vi "UNI_MAGFileToData.vi"(0 "spreadsheetData":string) -> (4 "names":string[](array[string]), 6 "settings":dbl[](array[numeric]) format="%.2f", 8 "polarities":i32[](array[numeric]), 10 "statuses":i32[](array[numeric]), 11 "allNames":bool, 12 "allSettings":bool, 13 "allPolarities":bool, 14 "allStatuses":bool, 15 "allRight":bool)   [LabVIEW 2014]
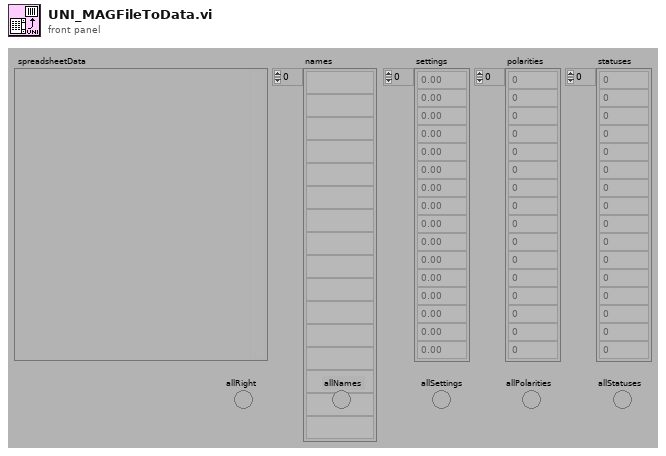
[diagram p1: front panel]
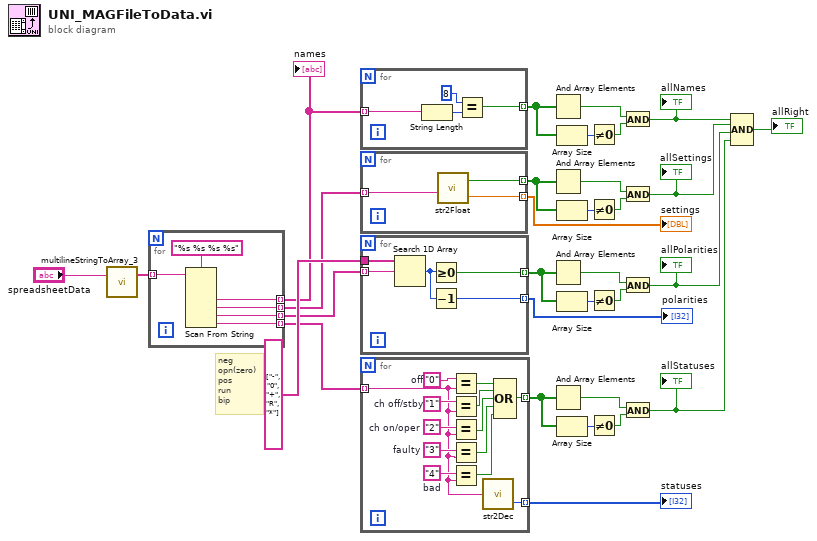
[diagram p0: block diagram]
diagram:
  # "neg\nopn(zero)\npos\nrun\nbip"
  n1 = call "multilineStringToArray_3.vi"("multilineString"="spreadsheetData") -> ("stringArray"=w15:string[])  [unwired: 1 in, 1 out]
  n2 = for {
    tunnel: w15 -> [w37] mode=indexing
    tunnel: [w35] -> w17 mode=indexing
    tunnel: [w34] -> w16 mode=indexing
    tunnel: [w33] -> w7 mode=indexing
    tunnel: [w32] -> w9 mode=indexing
    n3 = Scan From String(format string="%s %s %s %s", input string=w37) -> (output 1=w35:string, output 2=w34:string, output 3=w33:string, output 4=w32:string)  [unwired: 6 in, 3 out]
  }
  "names" <- w17
  n4 = for {
    tunnel: w17 -> [w41] mode=indexing
    tunnel: [w38] -> w19 mode=indexing
    n5 = String Length(string=w41) -> (length=w40:i32)
    n6 = Equal?(x=8, y=w40) -> (x = y?=w38:bool)
  }
  n7 = for {
    tunnel: w16 -> [w44] mode=indexing
    tunnel: [w43] -> w30 mode=indexing
    tunnel: [w42] -> w18 mode=indexing
    n8 = call "str2Float.vi"("string"=w44) -> ("is a floating"=w43:bool, "number"=w42:dbl)
  }
  "settings" <- w18
  n9 = for {
    tunnel: [w47] -> w24 mode=indexing
    tunnel: string[] ["-", "0", "+", "R", "*"] -> [w49]
    tunnel: w7 -> [w48] mode=indexing
    tunnel: [w45] -> w6 mode=indexing
    n10 = Search 1D Array(1D array=w49, element=w48) -> (index of element=w46:i32)  [unwired: 1 in]
    n11 = Greater Or Equal To 0?(x=w46) -> (x >= 0?=w47:bool)
    n12 = Decrement(x=w46) -> (x-1=w45:i32)
  }
  "polarities" <- w6
  n13 = for {
    tunnel: w9 -> [w51] mode=indexing
    tunnel: [w50] -> w12 mode=indexing
    tunnel: [w62] -> w8 mode=indexing
    w52 = "0"  # off
    w53 = "1"  # ch off/stby
    w54 = "2"  # ch on/oper
    w58 = "3"  # faulty
    w60 = "4"  # bad
    n14 = Equal?(x=w52, y=w51) -> (x = y?=w55:bool)
    n15 = Equal?(x=w53, y=w51) -> (x = y?=w56:bool)
    n16 = Equal?(x=w54, y=w51) -> (x = y?=w57:bool)
    n17 = Equal?(x=w58, y=w51) -> (x = y?=w59:bool)
    n18 = Equal?(x=w60, y=w51) -> (x = y?=w61:bool)
    n19 = call "str2Dec.vi"("string"=w51) -> ("number"=w62:i32)  [unwired: 1 out]
    n20 = Compound Arithmetic op=OR(w55, w56, w57, w59, w61) -> (w50:bool)
  }
  "statuses" <- w8
  n21 = And Array Elements(Boolean array=w19) -> (logical AND=w21:bool)
  n22 = And Array Elements(Boolean array=w30) -> (logical AND=w28:bool)
  n23 = And Array Elements(Boolean array=w24) -> (logical AND=w23:bool)
  n24 = And Array Elements(Boolean array=w12) -> (logical AND=w13:bool)
  n25 = Array Size(array=w19) -> (size(s)=w20:i32)
  n26 = Array Size(array=w30) -> (size(s)=w29:i32)
  n27 = Array Size(array=w24) -> (size(s)=w25:i32)
  n28 = Array Size(array=w12) -> (size(s)=w11:i32)
  n29 = Not Equal To 0?(x=w20) -> (x != 0?=w22:bool)
  n30 = Not Equal To 0?(x=w29) -> (x != 0?=w27:bool)
  n31 = Not Equal To 0?(x=w25) -> (x != 0?=w26:bool)
  n32 = Not Equal To 0?(x=w11) -> (x != 0?=w10:bool)
  n33 = And(x=w21, y=w22) -> (x .and. y?=w5:bool)
  "allNames" <- w5
  n34 = And(x=w28, y=w27) -> (x .and. y?=w4:bool)
  "allSettings" <- w4
  n35 = And(x=w23, y=w26) -> (x .and. y?=w3:bool)
  "allPolarities" <- w3
  n36 = And(x=w13, y=w10) -> (x .and. y?=w2:bool)
  "allStatuses" <- w2
  n37 = Compound Arithmetic op=AND(w5, w4, w3, w2) -> (→"allRight":bool)
